vi "merFISH_photobleaching_dialog_box.vi"(3 "error in":errorcluster, 4 "merFISH mode":u16, 5 "Injection procedure empty?":bool) -> (0 "error out":errorcluster, 2 "Which experiment?":T1(ring)=enum."Single ROIs & injections")   [LabVIEW 2015]
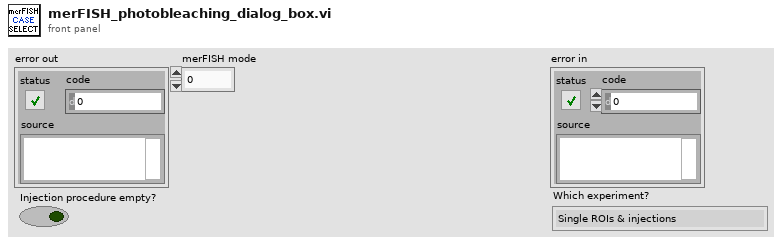
[diagram p1: front panel]
types:
  T1 = enum16{"Single ROIs & no injection", "Single ROIs & injections", "Embryos & no injection", "Embryos & injections"}
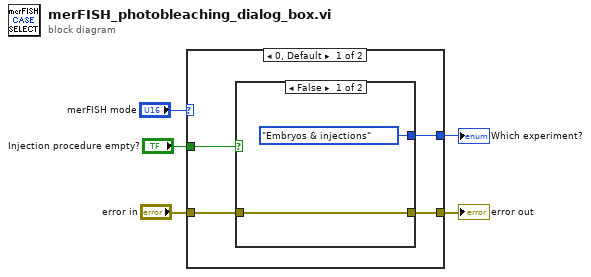
[diagram p0: block diagram]
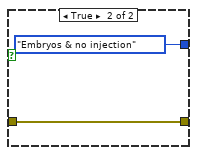
[diagram p2: hidden frame]
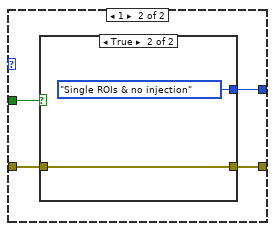
[diagram p3: hidden frame]
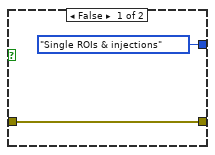
[diagram p4: hidden frame]
diagram:
  n1 = case shown="0, Default" "merFISH mode" {
    tunnel: "Injection procedure empty?" -> [w9 w15]
    tunnel: "error in" -> [w8 w16]
    tunnel: [w7 w17] -> w3
    tunnel: [w6 w14] -> w1
    frame 0, Default {
      n2 = case shown="False" w9 {
        tunnel: w8 -> [w11 w13]
        tunnel: [w11 w13] -> w7
        tunnel: [T1."Embryos & injections" ("Which experiment?") T1."Embryos & no injection" ("Which experiment?")] -> w6
        frame False {
        }
        frame True {
        }
      }
    }
    frame 1 {
      n3 = case shown="True" w15 {
        tunnel: w16 -> [w19 w21]
        tunnel: [w19 w21] -> w17
        tunnel: [T1."Single ROIs & injections" ("Which experiment?") T1."Single ROIs & no injection" ("Which experiment?")] -> w14
        frame False {
        }
        frame True {
        }
      }
    }
  }
  "error out" <- w3
  "Which experiment?" <- w1
